vi "Send Request To Execution Engine.vi"(0 "Request Message":string, 5 "Request Header":string, 7 "Request Content Type":i32(ring) items=["Info", "Warning", "Error", "Action"], 11 "error in":errorcluster) -> (15 "error out":errorcluster)   [LabVIEW 2023, in "RFFixtureCharact.Public.lvlib"]
uses:
  RFFixtureCharact.Public.lvlib
  Common/RFCalAndFixtureCharact.Common.lvlib
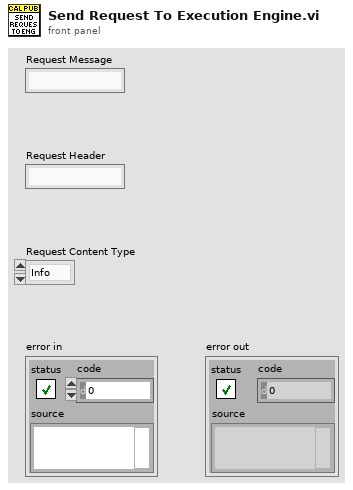
[diagram p1: front panel]
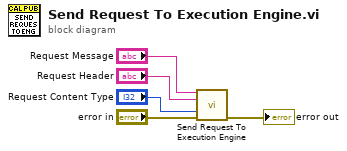
[diagram p0: block diagram]
diagram:
  n1 = call "Send Request To Execution Engine.vi"("Request Message"="Request Message", "Request Header"="Request Header", "Request Content Type"="Request Content Type", "error in (no error)"="error in") -> ("error out"=→"error out":errorcluster)  [unwired: 10 in, 1 out]
